vi "Read Attributes.vi"(11 "Verify and Check-in Msg":refnum<class "Verify and Check-in Msg.lvclass">) -> (2 "Payload":T1)   [LabVIEW 2023, in "Guest Manager UI.lvlib" / "Verify and Check-in Msg.lvclass"]
uses:
  Verify and Check-in Msg.lvclass
  Verify and Check-in Msg.lvclass/Verify and Check-in Msg.ctl
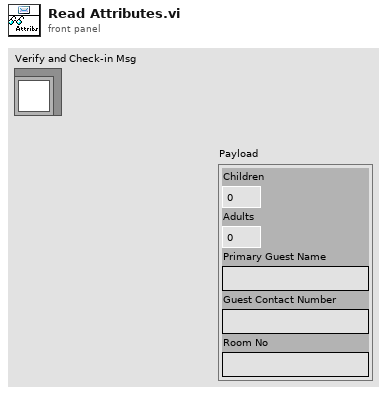
[diagram p1: front panel]
types:
  T1 = cluster{"Children":u32, "Adults":u32, "Primary Guest Name":string, "Guest Contact Number":string, "Room No":string}
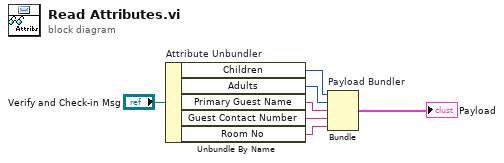
[diagram p0: block diagram]
diagram:
  n1 = Unbundle By Name "Attribute Unbundler"("Verify and Check-in Msg") -> ("Children"=w5:u32, "Adults"=w4:u32, "Primary Guest Name"=w3:string, "Guest Contact Number"=w2:string, "Room No"=w1:string)
  n2 = Bundle "Payload Bundler"("Children"=w5, "Adults"=w4, "Primary Guest Name"=w3, "Guest Contact Number"=w2, "Room No"=w1) -> (→"Payload":T1)  [unwired: 1 in]
